vi "App Version.vi"() -> (7 "App Version String":string)   [LabVIEW 2020, in "Builder Core.lvlib"]
uses:
  Builder Core.lvlib
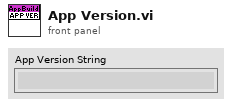
[diagram p1: front panel]
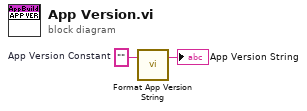
[diagram p0: block diagram]
diagram:
  w1 = ""  # App Version Constant
  n1 = call "Format App Version String.vi"("App Version String in"=w1) -> ("App Version String"=→"App Version String":string)  [unwired: 2 in]
